vi "Print Label.vi"() -> ()   [LabVIEW 2016]
uses:
  Control/state.ctl
  Control/ITEM_CLUSTER.ctl
  Control/Label data.ctl
  <vilib>/addons/database/Connection.llb/DB Tools Open Connec (Path).vi
  <vilib>/addons/database/_DB Variant To Data/Database Variant To Data.xnode
  <vilib>/addons/database/NI_Database_API.lvlib
panel:
  out "Min":string
  out "Max":string
  in  "Lot Maker":string
  out "Location":string
  out "Maker Code":string
  in  "BUTTON_EXIT":bool
  in  "BUTTON_PRINT":bool
  in  "Quantity":i32
  out "Lot Size":i32
  out "Unit":string
  out "Item Code (F3)":string
  in  "Part No.(F2)":string
  in  "Barcode (F1)":string
  out "Offset":i32
  out "Length":i32
  in  "Maker":string(combo)
  in  "Part Name":string(combo)
  in  "Product":string(combo)
  in  "ECODE":string
  in  "Invoice Date":timestamp format="%<%d/%m/%Y>T"
  in  "Invoice No.":string
  # "PRINT LABEL"
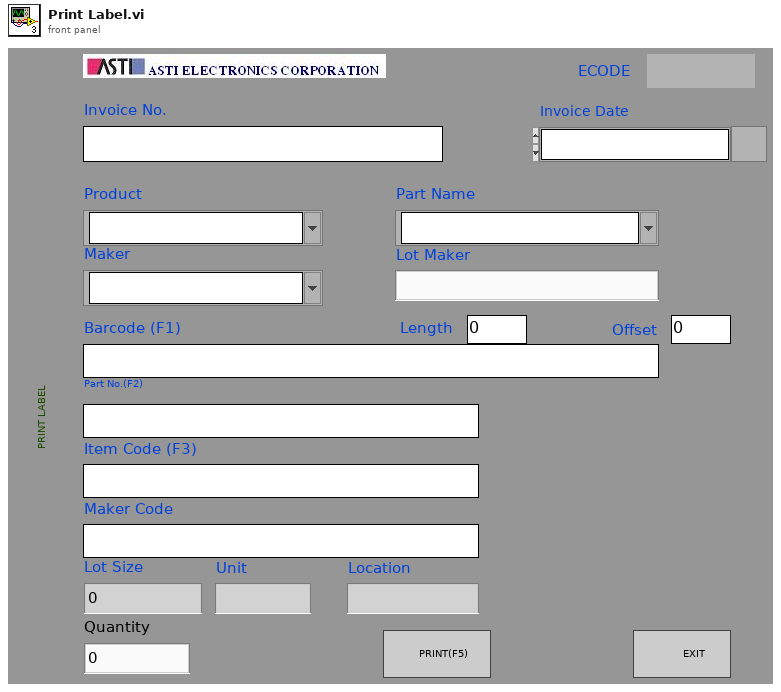
[diagram p1: front panel]
types:
  T1 = typedef "state.ctl" = enum16{"Initial", "Run", "Idle", "Exit"}
  T2 = typedef "NI_Database_API.lvlib/Conn ObjectReference.ctl" = refnum<k1>
  T3 = cluster{"Quantity":i32, "Offset":i32, "Length":i32}
  T4 = cluster{"MAKER":string, "PRODUCT":string, "PART NAME":string}
  T5 = cluster{"ECODE":string, "Barcode(F1)":string, "Lot Maker":string, "Part No.(F2)":string, "invoice No.":string, "Invoice Date":timestamp}
  T6 = typedef "ITEM_CLUSTER.ctl" = cluster{"PRODUCT":string, "ITEM_CODE":string, "PART_NAME":string, "MAKER":string, "PART_NO":string, "LOT_SIZE":string, "UNIT":string, "LENGTH-OFFSET":string, "BARCODE":string, "PROCESS":string, "INVENTORY_LOCAL":string, "TARE":string, "SAMPLE":string, "WARNING":string}
  T7 = typedef "Label data.ctl" = cluster{"Item Code":string, "ECode":string, "Part No.":string, "Maker":string, "Quantity":string, "Location":string, "Product":string, "Invoice No":string, "Invoice Date":string, "Lot maker":string}
  T8 = cluster{i32, "INVENTORY_LOCAL":string, "UNIT":string, "MAKER":string, "ITEM_CODE":string}
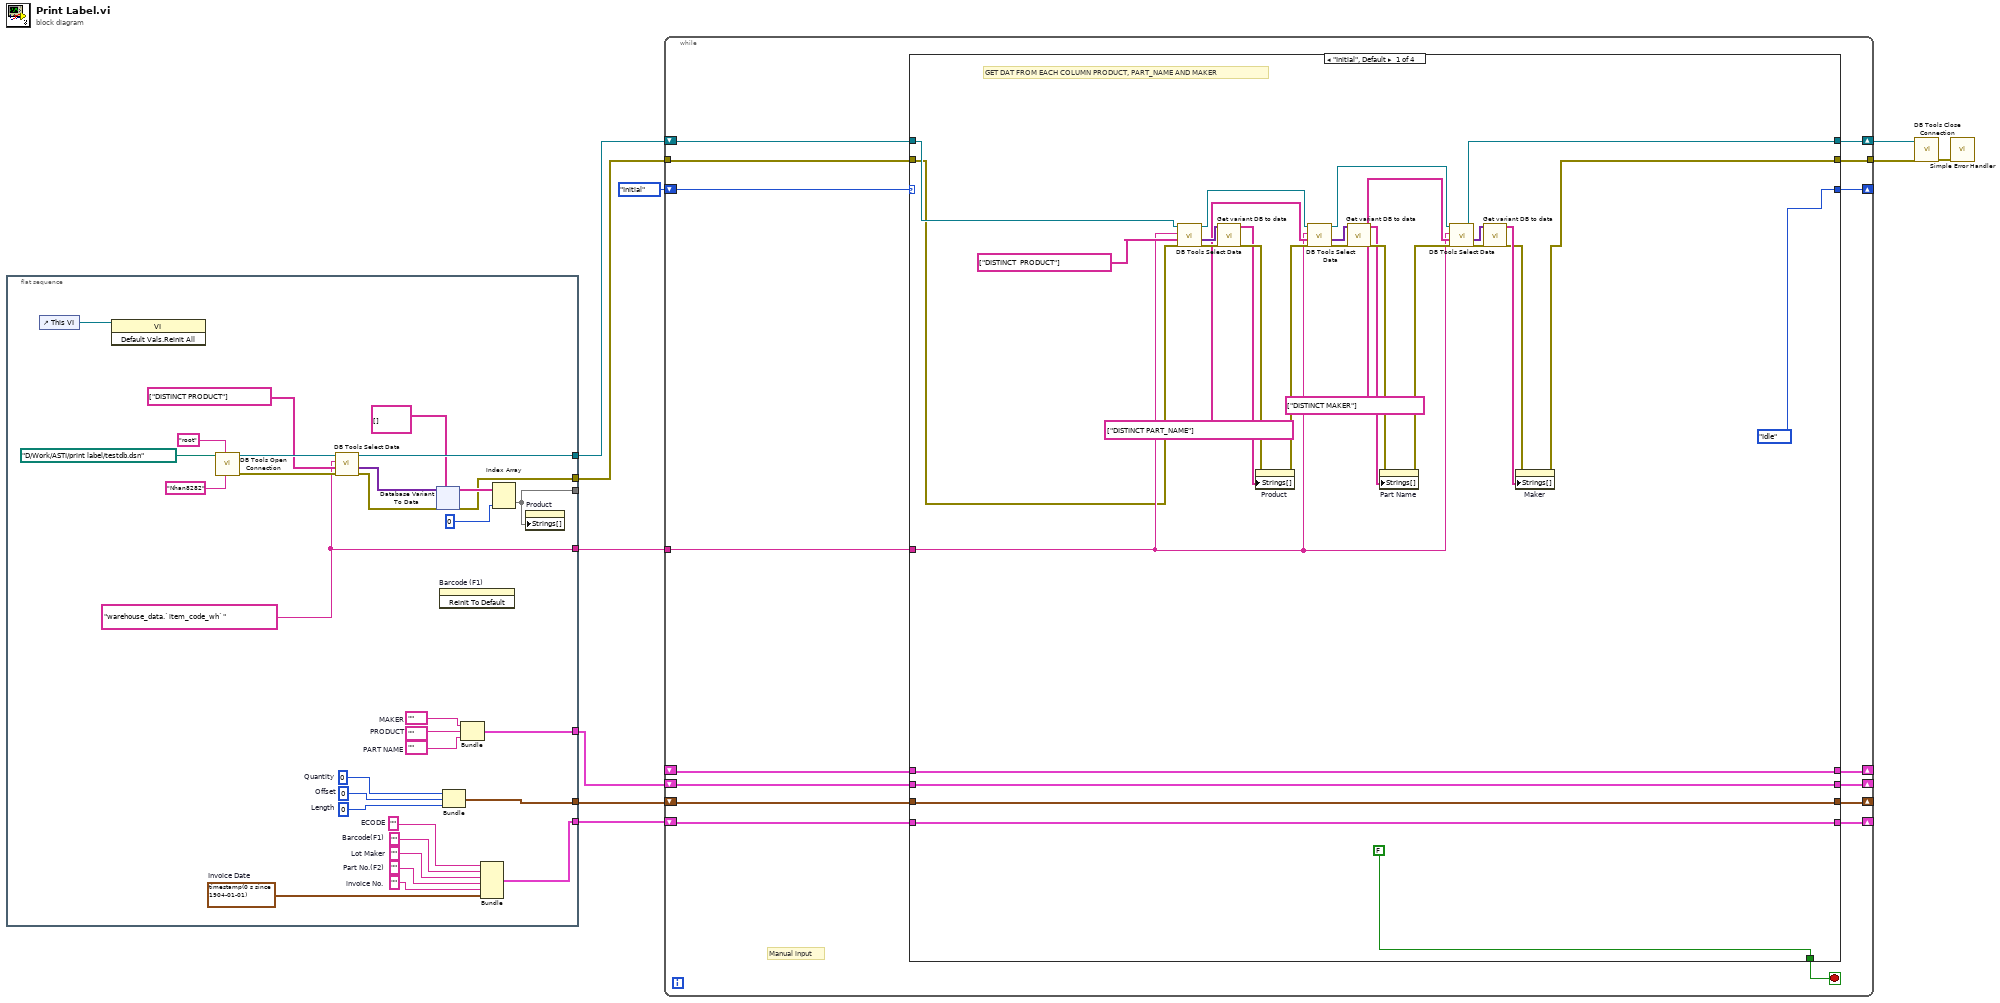
[diagram p0: block diagram]
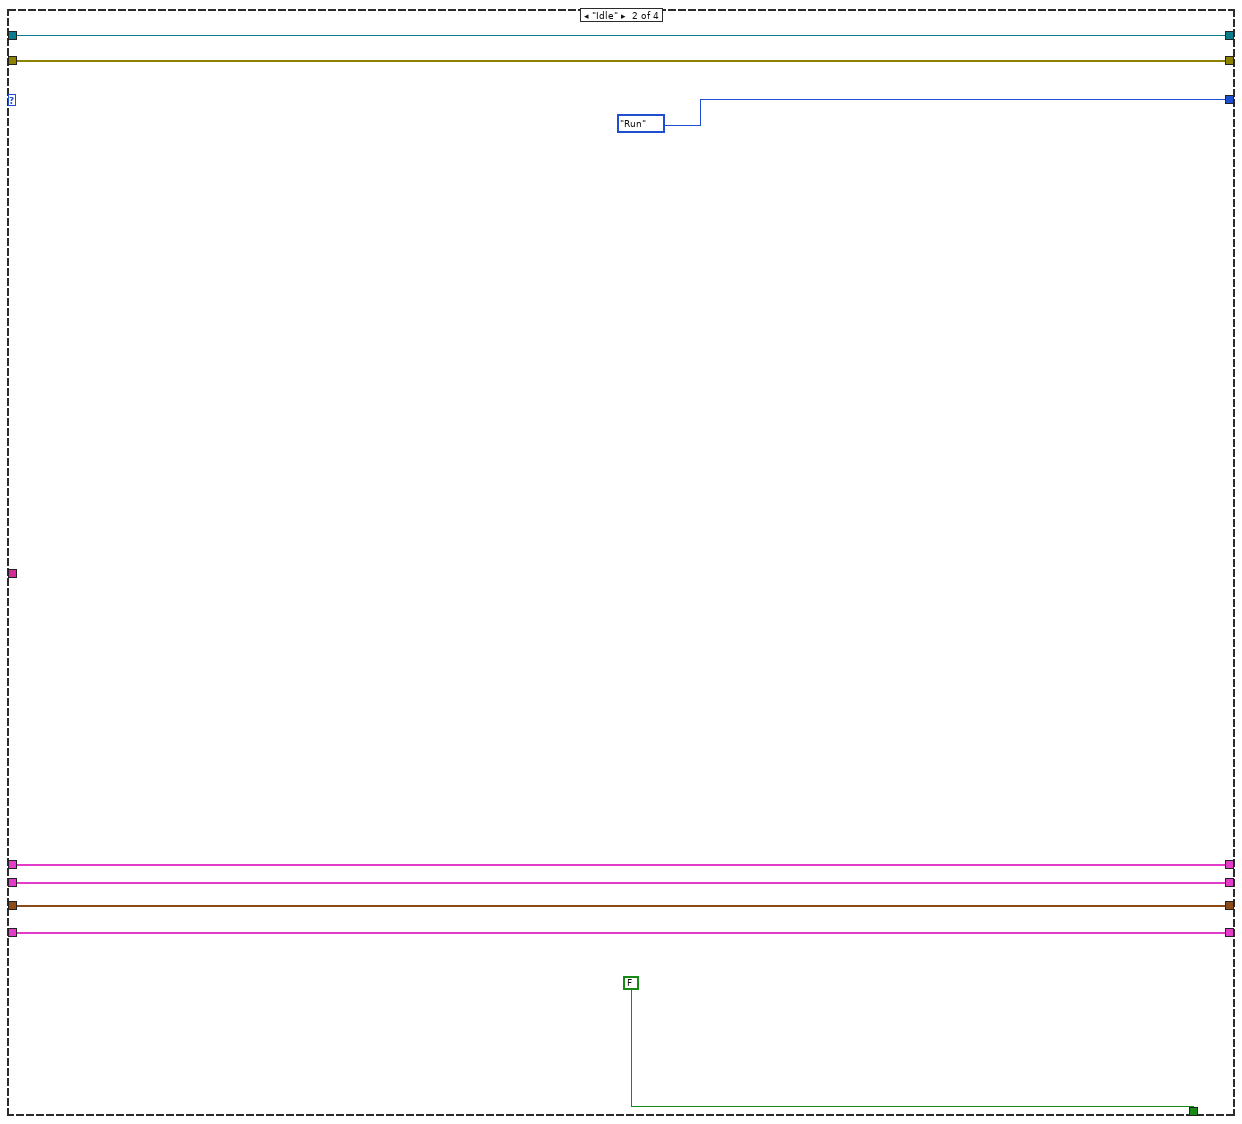
[diagram p2: hidden frame]
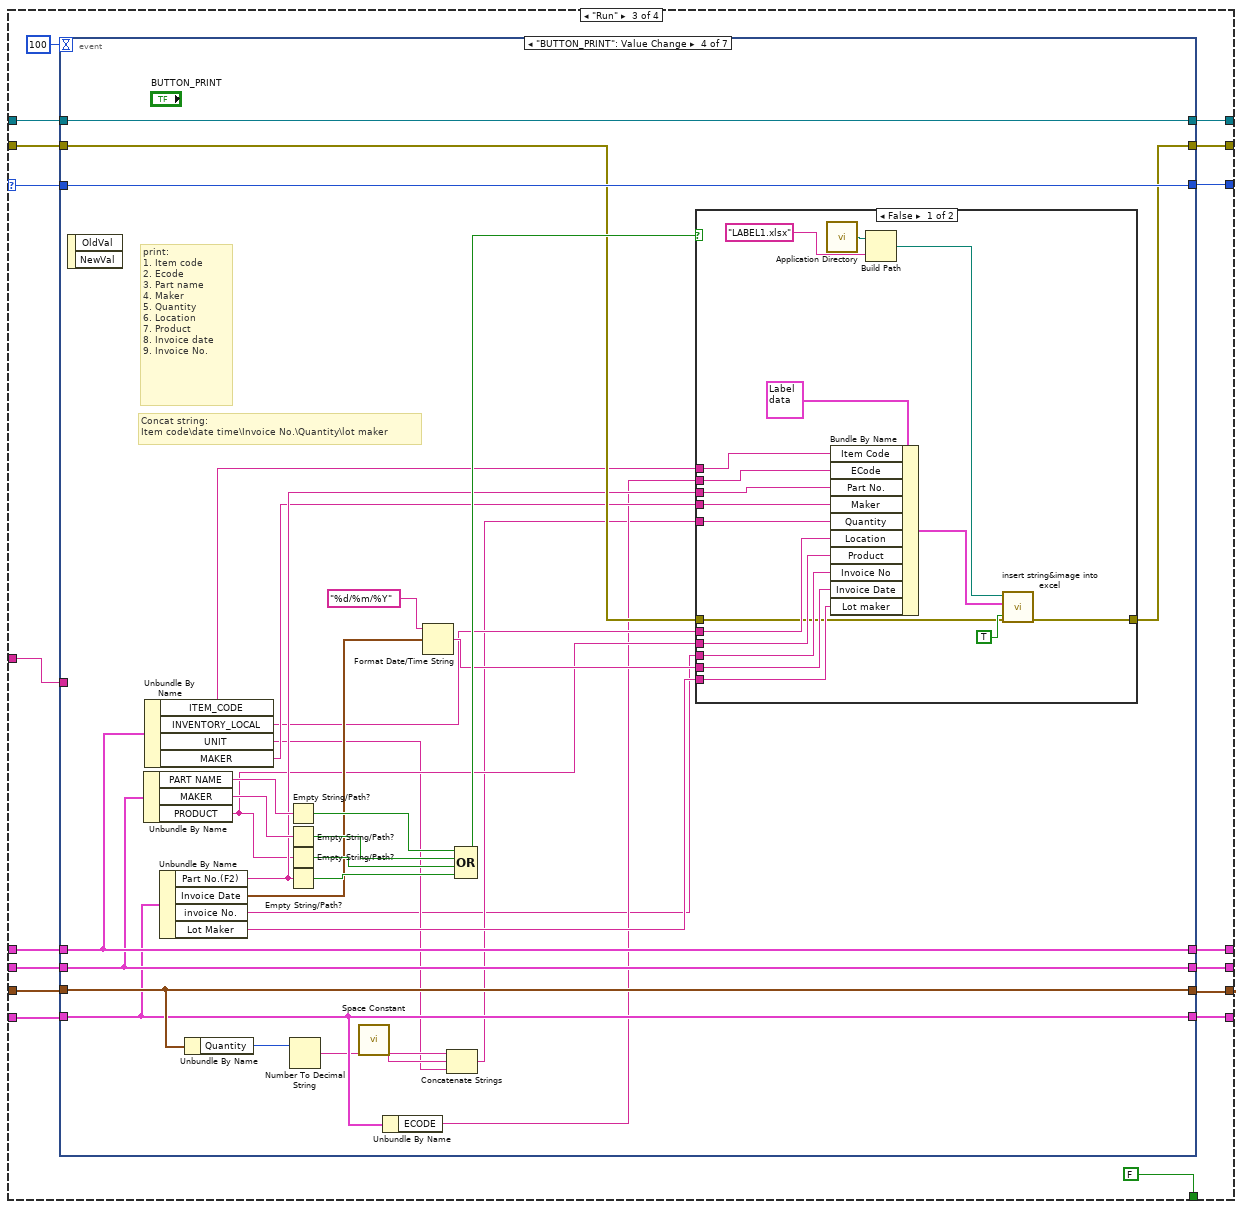
[diagram p3: hidden frame]
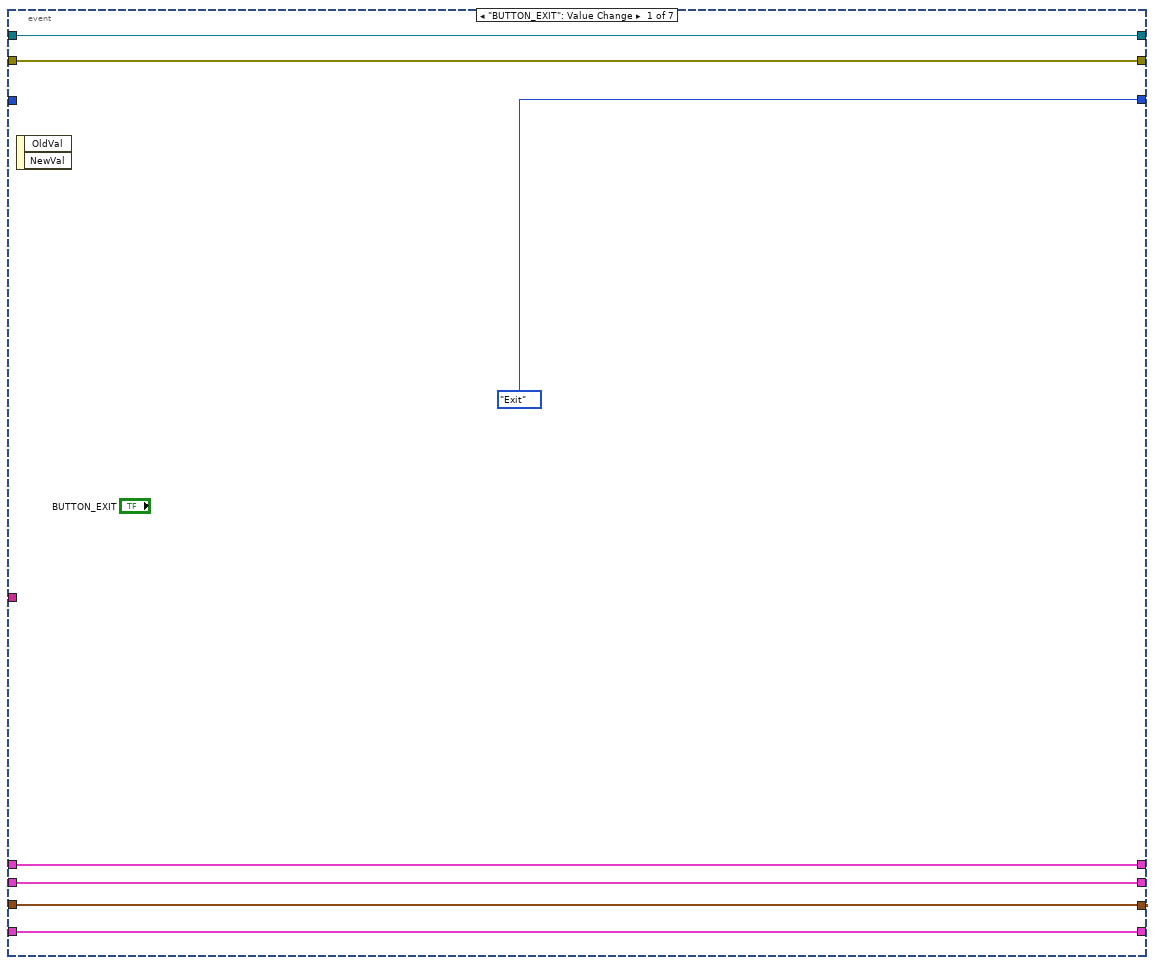
[diagram p4: hidden frame]
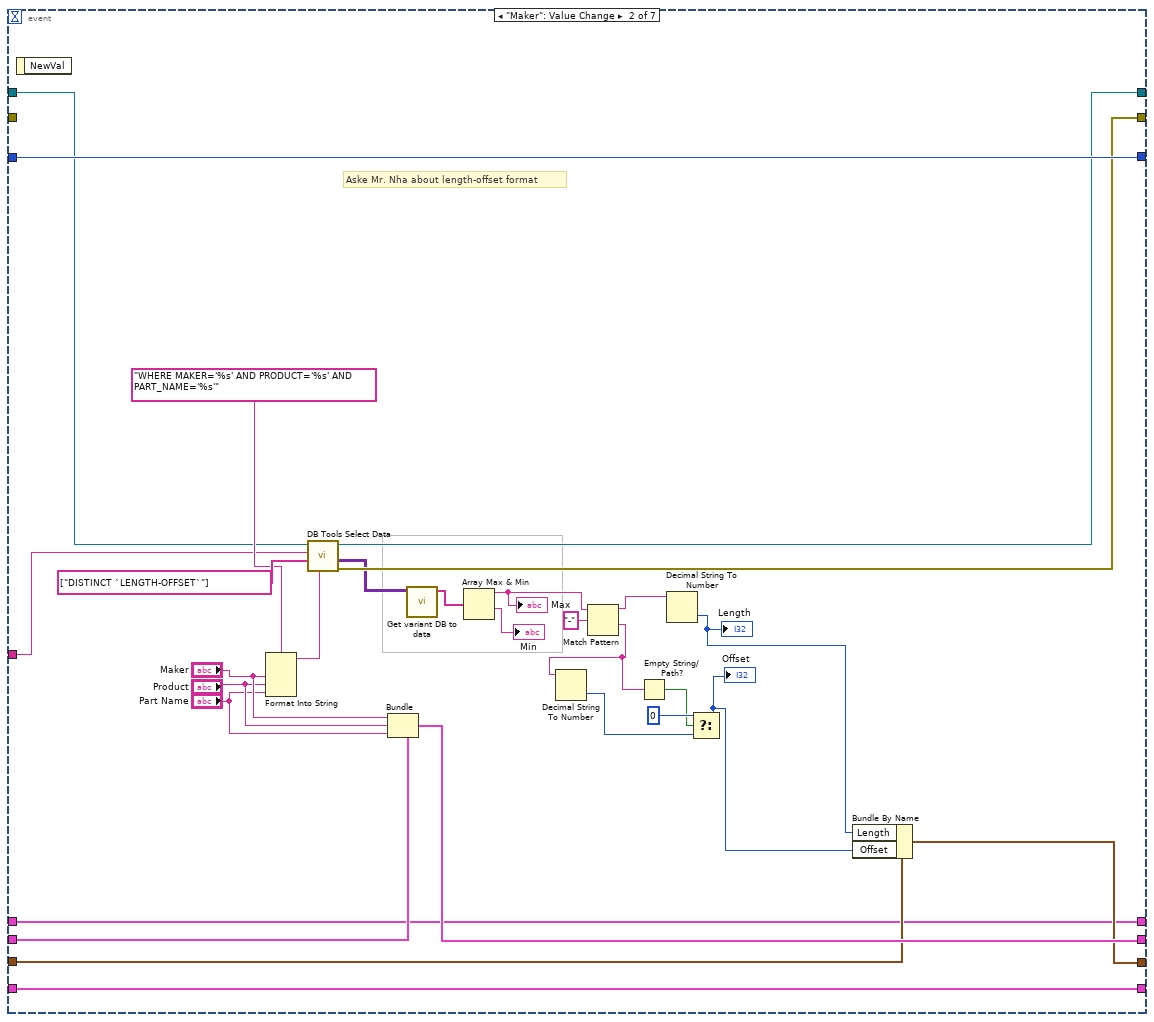
[diagram p5: hidden frame]
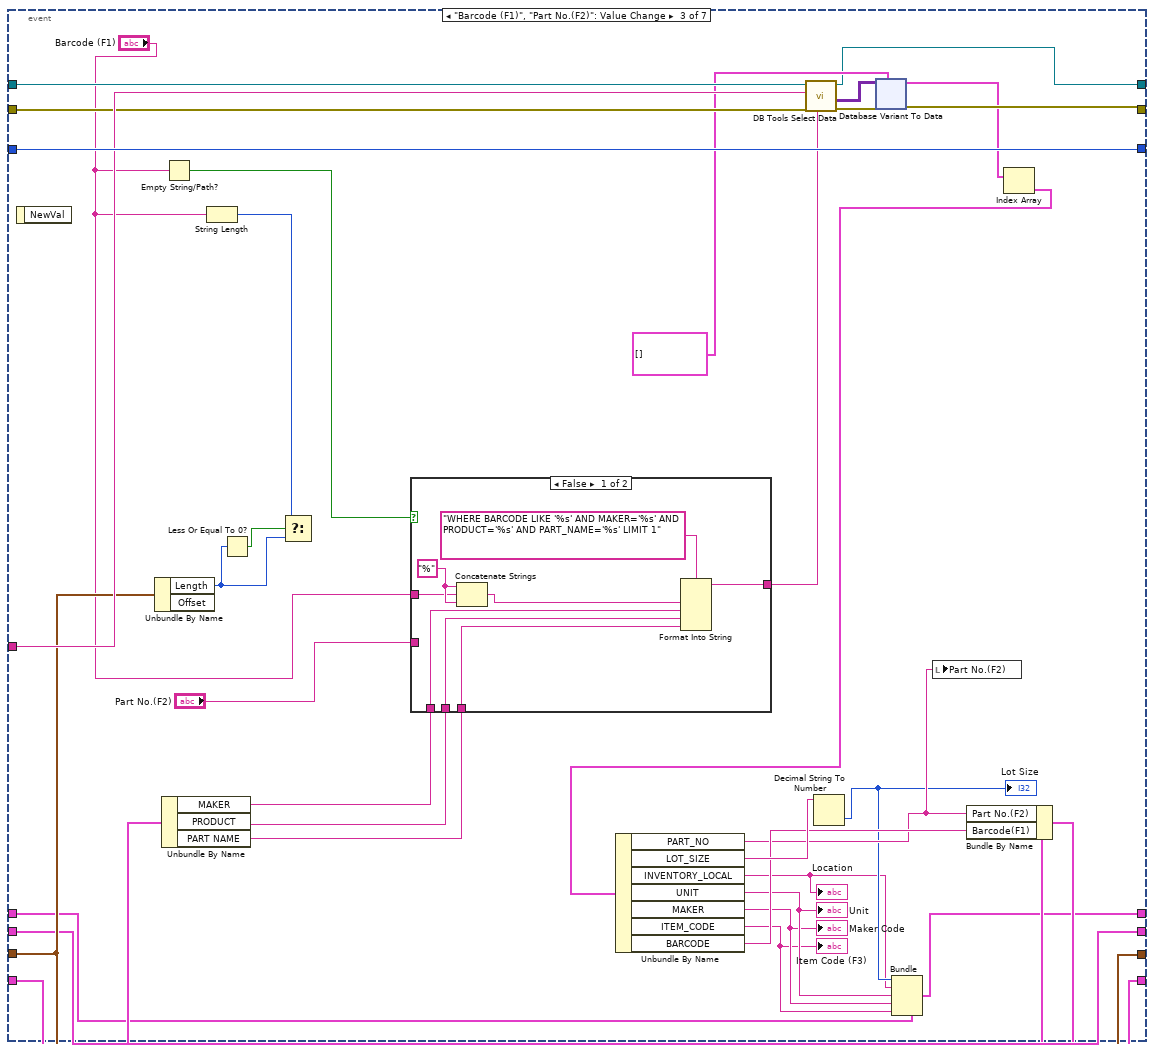
[diagram p6: hidden frame]
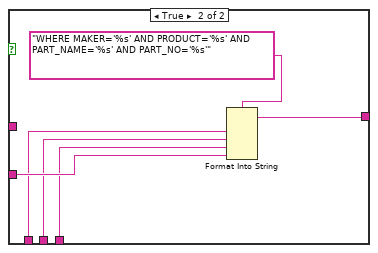
[diagram p7: hidden frame]
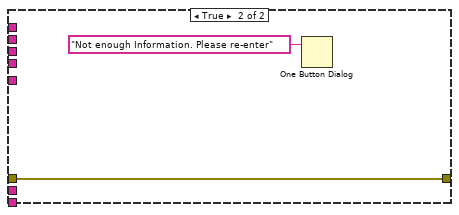
[diagram p8: hidden frame]
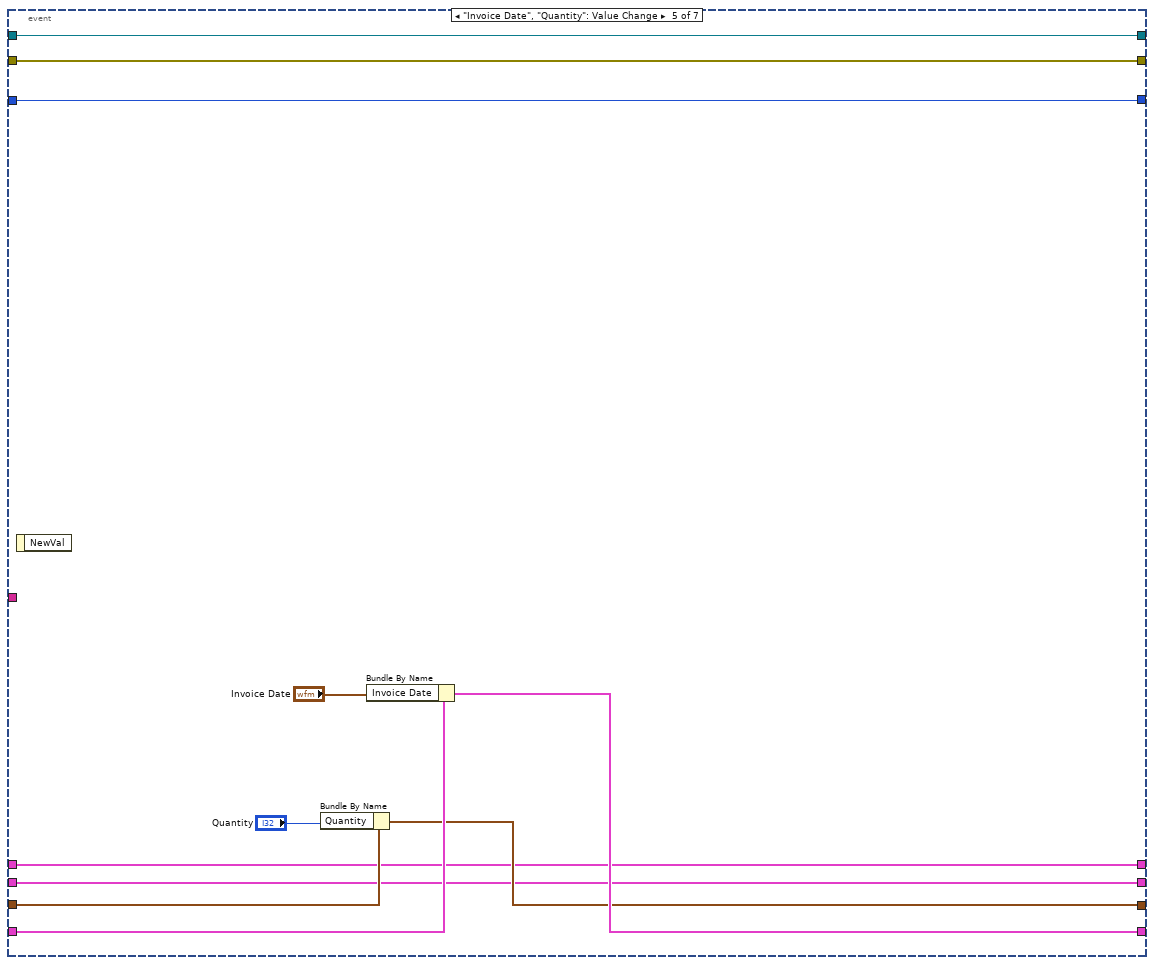
[diagram p9: hidden frame]
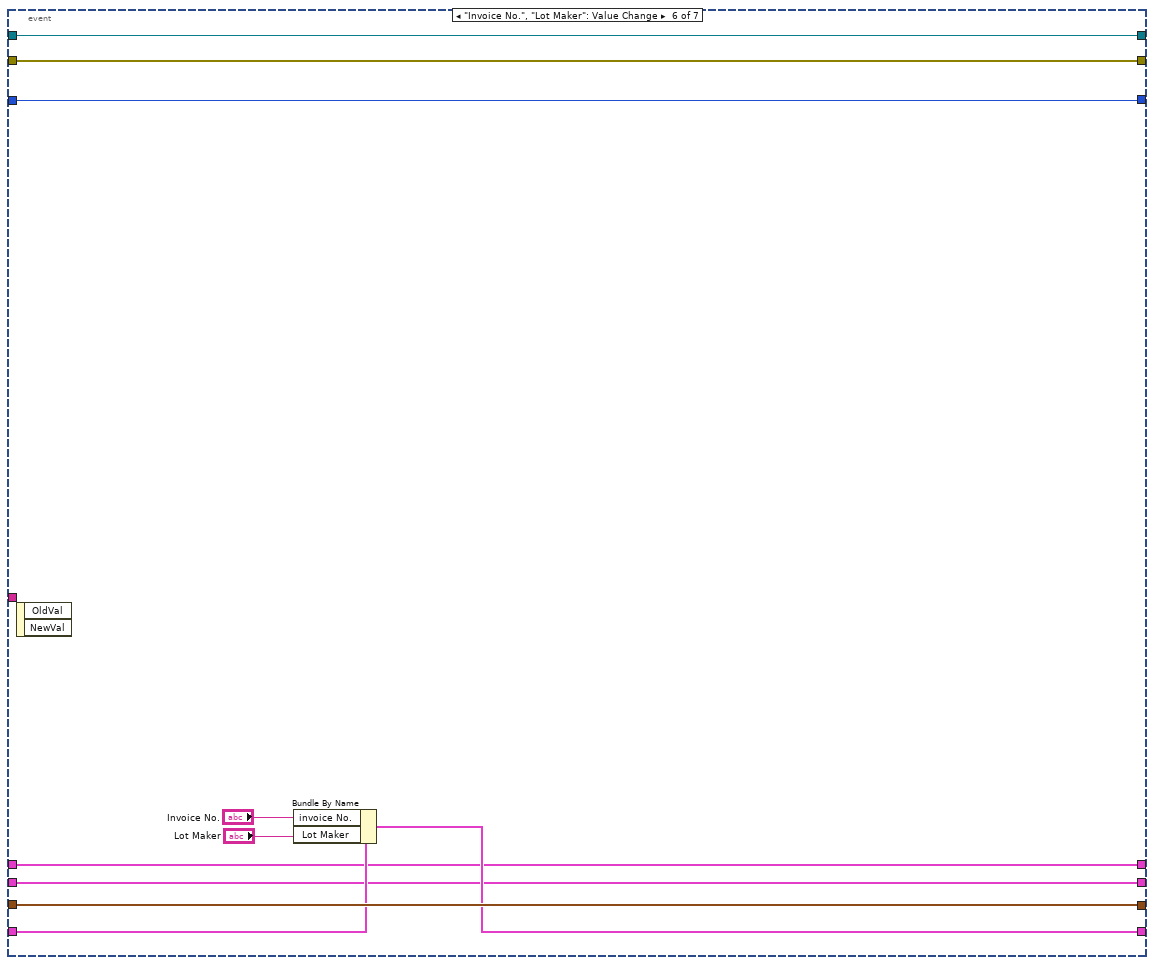
[diagram p10: hidden frame]
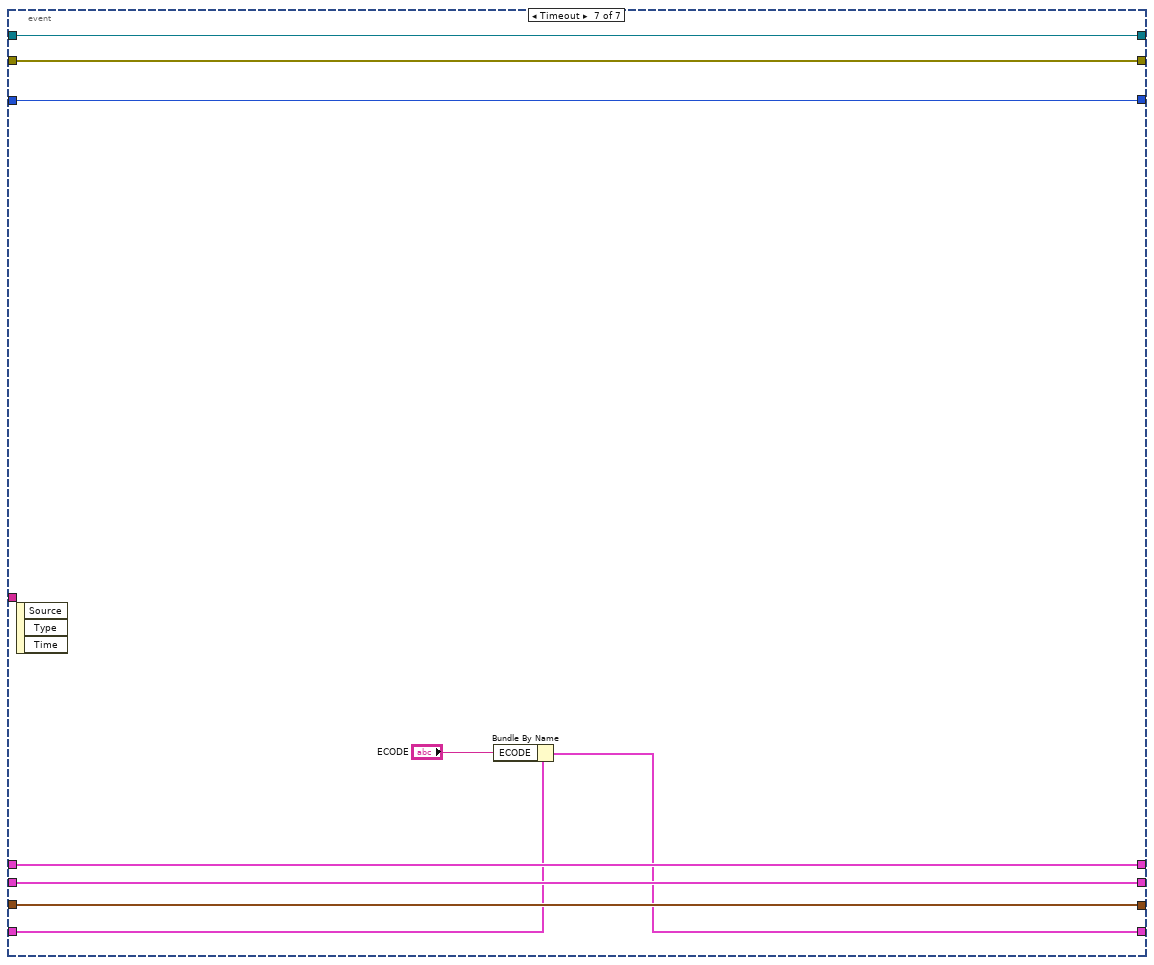
[diagram p11: hidden frame]
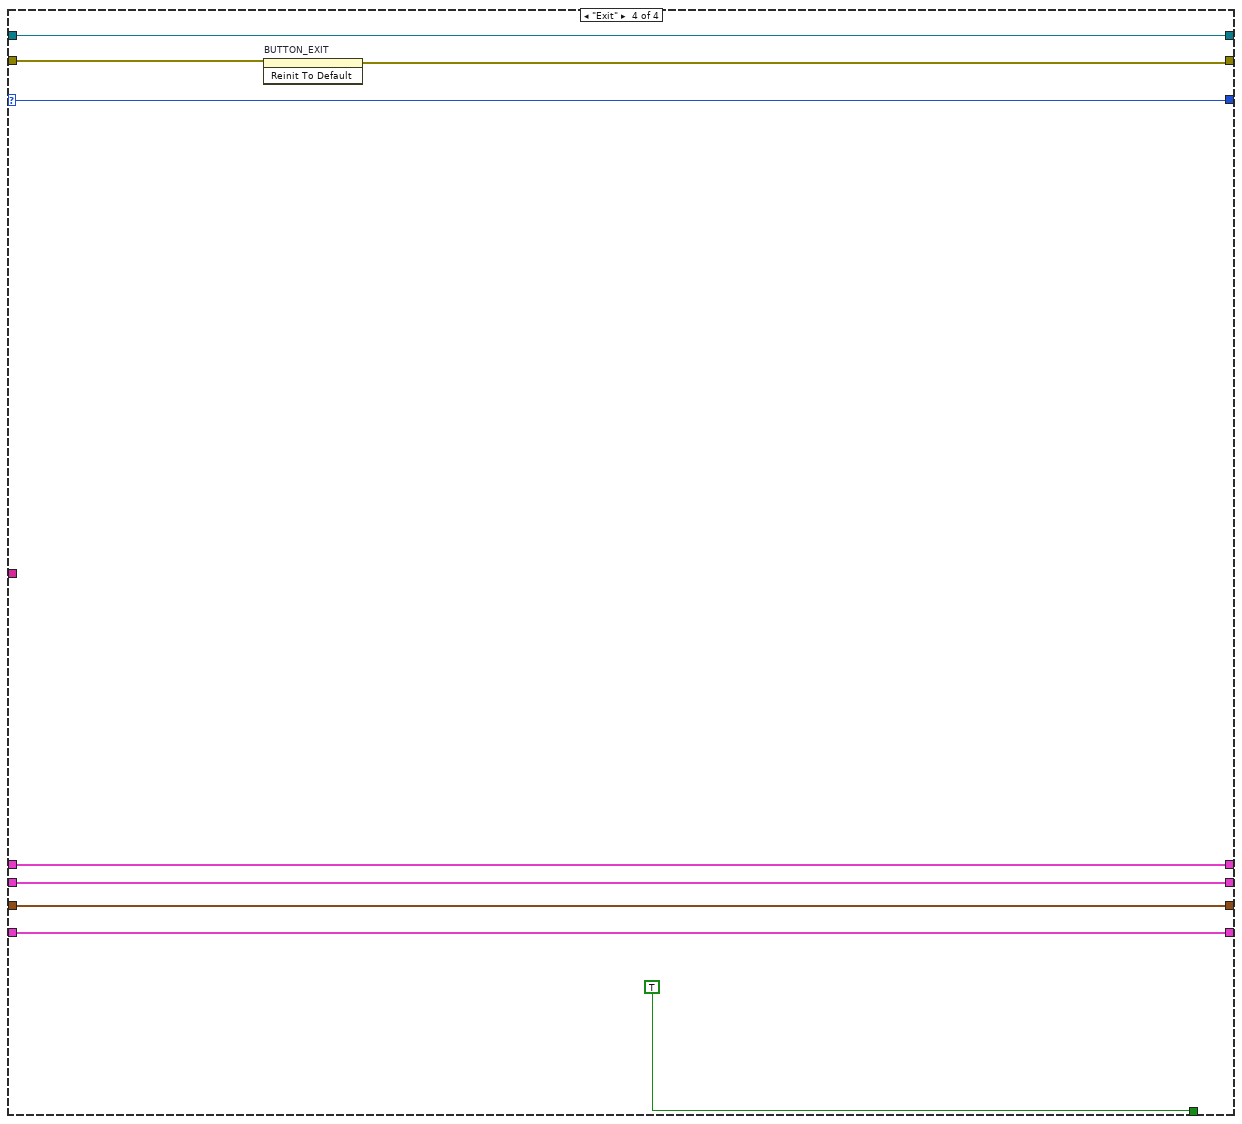
[diagram p12: hidden frame]
diagram:
  n1 = flat-sequence {
    tunnel: [w39] -> w8
    tunnel: [w24] -> w10
    tunnel: [w33] -> w3
    tunnel: [w31] -> w6
    tunnel: [w27] -> _
    tunnel: [w26] -> w2
    tunnel: [w12] -> w1
    frame #0 {
      w11 = ""  # ECODE
      w13 = ""  # PART NAME
      w14 = ""  # PRODUCT
      w15 = ""  # MAKER
      w16 = 0  # Quantity
      w20 = ""  # invoice No.
      w19 = ""  # Part No.(F2)
      w18 = ""  # Lot Maker
      w17 = ""  # Barcode(F1)
      w21 = timestamp(0 s since 1904-01-01)  # Invoice Date
      w22 = 0  # Length
      w23 = 0  # Offset
      w26 = "warehouse_data.`item_code_wh`"
      n2 = control-ref of="This VI"() -> (w25:refnum<vi>)
      n3 = invoke class="VI" method="Default Vals.Reinit All"(reference=w25) -> ()  [unwired: 2 in, 3 out]
      n4 = call-poly <vilib>:"DB Tools Open Connection.vi"("password"="Nhan8282" ("userID"), "userID"="root", "connection information"=path "D:/Work/ASTI/print label/testdb.dsn") -> ("error out"=w40:errorcluster, "connection reference"=w41:T2)  [unwired: 5 in]
      n5 = call <vilib>:"DB Tools Select Data.vi"("error in (no error)"=w40, "columns"=string[] ["DISTINCT PRODUCT"], "table"=w26, "connection reference"=w41) -> ("error out"=w32:errorcluster, "data"=w38:variant[][], "connection reference out"=w39:T2)  [unwired: 2 in]
      n6 = xnode "Database Variant To Data"("database variant"=w38, "error in (no error)"=w32, "type"=string[][] []) -> ("data"=w35:string[][], "error out"=w31:errorcluster)
      n7 = invoke on="Barcode (F1)" class="Str" method="Reinit To Default"() -> ()  [unwired: 3 in, 3 out]
      n8 = Bundle("Quantity"=w16, "Offset"=w23, "Length"=w22) -> (w24:T3)  [unwired: 1 in]
      n9 = Bundle("MAKER"=w15, "PRODUCT"=w14, "PART NAME"=w13) -> (w12:T4)  [unwired: 1 in]
      n10 = Bundle("ECODE"=w11, "Barcode(F1)"=w17, "Lot Maker"=w18, "Part No.(F2)"=w19, "invoice No."=w20, "Invoice Date"=w21) -> (w33:T5)  [unwired: 1 in]
      n11 = Index Array(array=w35, index (col)=0 ("index (row)")) -> (element=w27:string[])  [unwired: 1 in]
      n12 = property on="Product" class="CmbBox"("Strings[]"=w27) -> ()  [unwired: 2 in, 2 out]
    }
  }
  n13 = while {
    shift-right: [w98] -> _
    shift-left: w10 -> [w99]
    shift-right: [w97] -> _
    shift-left: w3 -> [w88]
    shift-right: [w100] -> _
    shift-left: state."Initial" ("Enum") -> [w101]
    shift-right: [w93] -> w7
    shift-left: w8 -> [w95]
    tunnel: w2 -> [w91]
    tunnel: w6 -> [w94]
    tunnel: [w92] -> w5
    shift-right: [w90] -> _
    shift-left: w1 -> [w89]
    shift-right: [w87] -> _
    shift-left: _ -> [w86]
    stop <- w96 stop-if-true
    # "Manual input"
    n14 = case shown="\"Initial\", Default" w101 {
      selector: w101 -> [_ _ w146 w773]
      tunnel: [state."Idle" ("Enum") state."Run" ("Enum") w155 w773] -> w100
      tunnel: w99 -> [w130 w139 w150 w775]
      tunnel: [w130 w139 w149 w775] -> w98
      tunnel: [w128 w138 w147 w774] -> w97
      tunnel: w88 -> [w128 w138 w148 w774]
      tunnel: [FALSE FALSE FALSE TRUE] -> w96
      tunnel: w95 -> [w108 w135 w154 w771]
      tunnel: w94 -> [w105 w134 w152 w770]
      tunnel: [w107 w135 w153 w771] -> w93
      tunnel: [w104 w134 w151 w769] -> w92
      tunnel: w91 -> [w106 _ w145 _]
      tunnel: [w103 w133 w144 w768] -> w90
      tunnel: w89 -> [w103 w133 w143 w768]
      tunnel: [w102 w132 w141 w767] -> w87
      tunnel: w86 -> [w102 w132 w140 w767]
      frame "Initial", Default {
        # "GET DAT FROM EACH COLUMN PRODUCT, PART_NAME AND MAKER"
        n15 = call <vilib>:"DB Tools Select Data.vi"("error in (no error)"=w105, "columns"=string[] ["DISTINCT  PRODUCT"], "table"=w106, "connection reference"=w108) -> ("error out"=w126:errorcluster, "data"=w125:variant[][], "connection reference out"=w122:T2)  [unwired: 2 in]
        n16 = call "Get variant DB to data.vi"("error in (no error)"=w126, "data in"=w125) -> ("error out"=w124:errorcluster, "data out"=w110:string[])  [unwired: 8 in]
        n17 = property on="Product" class="CmbBox"(error in=w124, "Strings[]"=w110) -> (error out=w123:errorcluster)  [unwired: 1 in, 1 out]
        n18 = call <vilib>:"DB Tools Select Data.vi"("error in (no error)"=w123, "columns"=string[] ["DISTINCT PART_NAME"], "table"=w106, "connection reference"=w122) -> ("error out"=w120:errorcluster, "data"=w119:variant[][], "connection reference out"=w109:T2)  [unwired: 2 in]
        n19 = call "Get variant DB to data.vi"("error in (no error)"=w120, "data in"=w119) -> ("error out"=w118:errorcluster, "data out"=w117:string[])  [unwired: 8 in]
        n20 = property on="Part Name" class="CmbBox"(error in=w118, "Strings[]"=w117) -> (error out=w116:errorcluster)  [unwired: 1 in, 1 out]
        n21 = call <vilib>:"DB Tools Select Data.vi"("error in (no error)"=w116, "columns"=string[] ["DISTINCT MAKER"], "table"=w106, "connection reference"=w109) -> ("error out"=w114:errorcluster, "data"=w113:variant[][], "connection reference out"=w107:T2)  [unwired: 2 in]
        n22 = call "Get variant DB to data.vi"("error in (no error)"=w114, "data in"=w113) -> ("error out"=w111:errorcluster, "data out"=w112:string[])  [unwired: 8 in]
        n23 = property on="Maker" class="CmbBox"(error in=w111, "Strings[]"=w112) -> (error out=w104:errorcluster)  [unwired: 1 in, 1 out]
      }
      frame "Idle" {
      }
      frame "Run" {
        n24 = event shown="[3] \"BUTTON_PRINT\": Value Change" {
          selector: _ -> [_ _ _ _ _ _ _]
          dyn-events: _ -> [_ _ _ _ _ _ _]
          timeout: 100 -> [_ _ _ _ _ _ _]
          tunnel: [state."Exit" ("Enum") w188 w227 w716 w747 w757 w766] -> w155
          tunnel: w154 -> [w162 w185 w222 w715 w746 w756 w765]
          tunnel: [w162 w187 w216 w715 w746 w756 w765] -> w153
          tunnel: [w161 w186 w217 w704 w745 w755 w764] -> w151
          tunnel: w152 -> [w161 _ w221 w705 w745 w755 w764]
          tunnel: [w160 w166 w213 w703 w741 w754 w763] -> w149
          tunnel: w150 -> [w160 w169 w213 w703 w742 w754 w763]
          tunnel: w148 -> [w159 w192 w202 w696 w744 w753 w759]
          tunnel: [w159 w192 w201 w696 w743 w752 w758] -> w147
          tunnel: w146 -> [_ w188 w227 w716 w747 w757 w766]
          tunnel: w145 -> [_ w184 w223 _ _ _ _]
          tunnel: [w158 w180 w205 w707 w738 w749 w762] -> w144
          tunnel: w143 -> [w158 w165 w205 w707 w738 w749 w762]
          tunnel: [w157 w164 w195 w708 w737 w748 w761] -> w141
          tunnel: w140 -> [w157 w164 w194 w708 w737 w748 w761]
          event "BUTTON_EXIT": Value Change {
            n25 = event-data() -> ()  [unwired: 1 in, 2 out]
          }
          event "Maker": Value Change {
            # "Aske Mr. Nha about length-offset format"
            n26 = event-data() -> ()  [unwired: 1 in, 1 out]
            n27 = Format Into String(format string="WHERE MAKER='%s' AND PRODUCT='%s' AND PART_NAME='%s'" ("condition"), "Maker", "Product", "Part Name") -> (resulting string=w189:string)  [unwired: 2 in, 1 out]
            n28 = call <vilib>:"DB Tools Select Data.vi"("condition"=w189, "columns"=string[] ["DISTINCT `LENGTH-OFFSET`"], "table"=w184, "connection reference"=w185) -> ("error out"=w186:errorcluster, "data"=w179:variant[][], "connection reference out"=w187:T2)  [unwired: 2 in]
            n29 = Bundle(cluster=w165, "MAKER"="Maker", "PRODUCT"="Product", "PART NAME"="Part Name") -> (w180:T4)
            n30 = call "Get variant DB to data.vi"("data in"=w179) -> ("data out"=w178:string[])  [unwired: 9 in, 1 out]
            n31 = Array Max & Min(array=w178) -> (max value=w176:string, min value=→"Min":string)  [unwired: 2 out]
            "Max" <- w176
            n32 = Match Pattern(string=w176, regular expression="-") -> (before substring=w174:string, after substring=w173:string)  [unwired: 1 in, 2 out]
            n33 = Decimal String To Number(string=w173) -> (number=w170:i32)  [unwired: 2 in, 1 out]
            n34 = Empty String/Path?(string/path=w173) -> (empty?=w171:bool)
            n35 = Decimal String To Number(string=w174) -> (number=w168:i32)  [unwired: 2 in, 1 out]
            "Length" <- w168
            n36 = Select(t=0, s=w171, f=w170) -> (s? t:f=w167:i32)
            "Offset" <- w167
            n37 = Bundle By Name(cluster=w169, "Length"=w168, "Offset"=w167) -> (w166:T3)
          }
          event "Barcode (F1)", "Part No.(F2)": Value Change {
            n38 = event-data() -> ()  [unwired: 1 in, 1 out]
            n39 = Unbundle By Name(w213) -> ("Length"=w212:i32)  [unwired: 1 out]
            n40 = Unbundle By Name(w205) -> ("MAKER"=w211:string, "PRODUCT"=w210:string, "PART NAME"=w209:string)
            n41 = Empty String/Path?(string/path="Barcode (F1)") -> (empty?=w214:bool)
            n42 = String Length(string="Barcode (F1)") -> (length=w225:i32)
            n43 = Less Or Equal To 0?(x=w212) -> (x <= 0?=w226:bool)
            n44 = Select(t=w225, s=w226, f=w212) -> ()  [unwired: 1 out]
            n45 = case shown="False" w214 {
              tunnel: [w676 w683] -> w224
              tunnel: "Part No.(F2)" -> [_ w684]
              tunnel: w211 -> [w675 w682]
              tunnel: w210 -> [w674 w681]
              tunnel: w209 -> [w673 w680]
              tunnel: "Barcode (F1)" -> [w672 _]
              frame False {
                w678 = "%"
                n46 = Concatenate Strings(w678, w672, w678) -> (w677:string)
                n47 = Format Into String(format string="WHERE BARCODE LIKE '%s' AND MAKER='%s' AND PRODUCT='%s' AND PART_NAME='%s' LIMIT 1" ("condition"), w677, w675, w674, w673) -> (resulting string=w676:string)  [unwired: 2 in, 1 out]
              }
              frame True {
                n48 = Format Into String(format string="WHERE MAKER='%s' AND PRODUCT='%s' AND PART_NAME='%s' AND PART_NO='%s'" ("condition"), w682, w681, w680, w684) -> (resulting string=w683:string)  [unwired: 2 in, 1 out]
              }
            }
            n49 = call <vilib>:"DB Tools Select Data.vi"("condition"=w224, "error in (no error)"=w221, "table"=w223, "connection reference"=w222) -> ("error out"=w220:errorcluster, "data"=w219:variant[][], "connection reference out"=w216:T2)  [unwired: 2 in]
            n50 = xnode "Database Variant To Data"("database variant"=w219, "error in (no error)"=w220, "type"=T6[] []) -> ("data"=w215:T6[], "error out"=w217:errorcluster)
            n51 = Index Array(array=w215) -> (element=w208:T6)  [unwired: 1 in]
            n52 = Unbundle By Name(w208) -> ("PART_NO"=w203:string, "LOT_SIZE"=w206:string, "INVENTORY_LOCAL"=w199:string, "UNIT"=w198:string, "MAKER"=w197:string, "ITEM_CODE"=w196:string, "BARCODE"=w204:string)
            "Item Code (F3)" <- w196
            "Unit" <- w198
            "Maker Code" <- w197
            "Location" <- w199
            n53 = Decimal String To Number(string=w206) -> (number=w200:i32)  [unwired: 2 in, 1 out]
            "Lot Size" <- w200
            n54 = Bundle(cluster=w194, w200, "INVENTORY_LOCAL"=w199, "UNIT"=w198, "MAKER"=w197, "ITEM_CODE"=w196) -> (w195:T8)
            n55 = local write "Part No.(F2)"(w203) -> ()
            n56 = Bundle By Name(cluster=w202, "Part No.(F2)"=w203, "Barcode(F1)"=w204) -> (w201:T5)
          }
          event "BUTTON_PRINT": Value Change {
            # "Concat string: \nItem code\\date time\\Invoice No.\\Quantity\\lot maker"
            # "print: \n1. Item code\n2. Ecode \n3. Part name\n4. Maker\n5. Quantity\n6. Location\n7. Product\n8. Invoice date\n9. Invoice No."
            n57 = event-data() -> ()  [unwired: 1 in, 2 out]
            n58 = Unbundle By Name(w707) -> ("PART NAME"=w710:string, "MAKER"=w709:string, "PRODUCT"=w692:string)
            n59 = Unbundle By Name(w708) -> ("ITEM_CODE"=w702:string, "INVENTORY_LOCAL"=w693:string, "UNIT"=w688:string, "MAKER"=w694:string)
            n60 = Unbundle By Name(w696) -> ("Part No.(F2)"=w695:string, "Invoice Date"=w701:timestamp, "invoice No."=w686:string, "Lot Maker"=w697:string)
            n61 = Unbundle By Name(w703) -> ("Quantity"=w698:i32)
            n62 = Empty String/Path?(string/path=w710) -> (empty?=w714:bool)
            n63 = Empty String/Path?(string/path=w709) -> (empty?=w713:bool)
            n64 = Empty String/Path?(string/path=w692) -> (empty?=w712:bool)
            n65 = Empty String/Path?(string/path=w695) -> (empty?=w711:bool)
            n66 = Number To Decimal String(number=w698) -> (decimal integer string=w690:string)  [unwired: 1 in]
            n67 = call <vilib>:"Space Constant.vi"() -> ("String"=w689:string)
            n68 = Unbundle By Name(w696) -> ("ECODE"=w691:string)
            n69 = Format Date/Time String(time format string (%c)="%d/%m/%Y", seconds (now)=w701) -> (date/time string=w699:string)  [unwired: 1 in]
            n70 = Concatenate Strings(w690, w689, w688) -> (w687:string)
            n71 = Compound Arithmetic op=OR(w714, w713, w712, w711) -> (w706:bool)
            n72 = case shown="False" w706 {
              tunnel: w705 -> [w718 w735]
              tunnel: [w717 w735] -> w704
              tunnel: w702 -> [w733 _]
              tunnel: w699 -> [w725 _]
              tunnel: w697 -> [w724 _]
              tunnel: w691 -> [w732 _]
              tunnel: w695 -> [w731 _]
              tunnel: w694 -> [w730 _]
              tunnel: w693 -> [w729 _]
              tunnel: w692 -> [w728 _]
              tunnel: w687 -> [w727 _]
              tunnel: w686 -> [w726 _]
              frame False {
                n73 = call <vilib>:"Application Directory.vi"() -> ("Application Directory"=w720:path)
                n74 = Bundle By Name(cluster=T7 {"Item Code"="Item code 1", "ECode"="Ecode", "Part No."="Part No. ", "Maker"="Maker", "Quantity"="Quantity", "Location"="Location", "Product"="Product", "Invoice No"="Invoice No", "Invoice Date"="Invoice Date", "Lot maker"="Invoice Date"} ("Item_Information"), "Item Code"=w733, "ECode"=w732, "Part No."=w731, "Maker"=w730, "Quantity"=w727, "Location"=w729, "Product"=w728, "Invoice No"=w726, "Invoice Date"=w725, "Lot maker"=w724) -> (w723:T7)
                n75 = Build Path(base path=w720, name or relative path="LABEL1.xlsx") -> (appended path=w719:path)
                n76 = call "insert string&image into excel.vi"("Print QR"=TRUE ("Print Button"), "error in"=w718, "Item_Information"=w723, "template Path"=w719) -> ("error out"=w717:errorcluster)  [unwired: 7 in]
              }
              frame True {
                n77 = One Button Dialog(message="Not enough Information. Please re-enter") -> ()  [unwired: 1 in, 1 out]
              }
            }
          }
          event "Invoice Date", "Quantity": Value Change {
            n78 = event-data() -> ()  [unwired: 1 in, 1 out]
            n79 = Bundle By Name(cluster=w742, "Quantity"="Quantity") -> (w741:T3)
            n80 = Bundle By Name(cluster=w744, "Invoice Date"="Invoice Date") -> (w743:T5)
          }
          event "Invoice No.", "Lot Maker": Value Change {
            n81 = event-data() -> ()  [unwired: 1 in, 2 out]
            n82 = Bundle By Name(cluster=w753, "invoice No."="Invoice No.", "Lot Maker"="Lot Maker") -> (w752:T5)
          }
          event Timeout {
            n83 = event-data() -> ()  [unwired: 1 in, 3 out]
            n84 = Bundle By Name(cluster=w759, "ECODE"="ECODE") -> (w758:T5)
          }
        }
      }
      frame "Exit" {
        n85 = invoke on="BUTTON_EXIT" class="Bool" method="Reinit To Default"(error in=w770) -> (error out=w769:errorcluster)  [unwired: 2 in, 2 out]
      }
    }
  }
  n86 = call <vilib>:"DB Tools Close Connection.vi"("error in (no error)"=w5, "connection reference"=w7) -> ("error out"=w4:errorcluster)  [unwired: 5 in]
  n87 = call <vilib>:"Simple Error Handler.vi"("error in (no error)"=w4) -> ()  [unwired: 4 in, 5 out]
